vi "001 planta emotelladora.vi"() -> ()   [LabVIEW 2019]
panel:
  in  "pos ampolla plena":dbl(slide) scale=0.0..100.0
  out "Horizontal Pointer Slide":dbl(slide) scale=0.0..100.0
  in  "dispensador":dbl(slide) scale=0.0..10.0
  out "Slide":dbl(slide) scale=0.0..10.0
  in  "pos ampolla buida":dbl(slide) scale=0.0..100.0
  out "Horizontal Pointer Slide 2":dbl(slide) scale=0.0..100.0
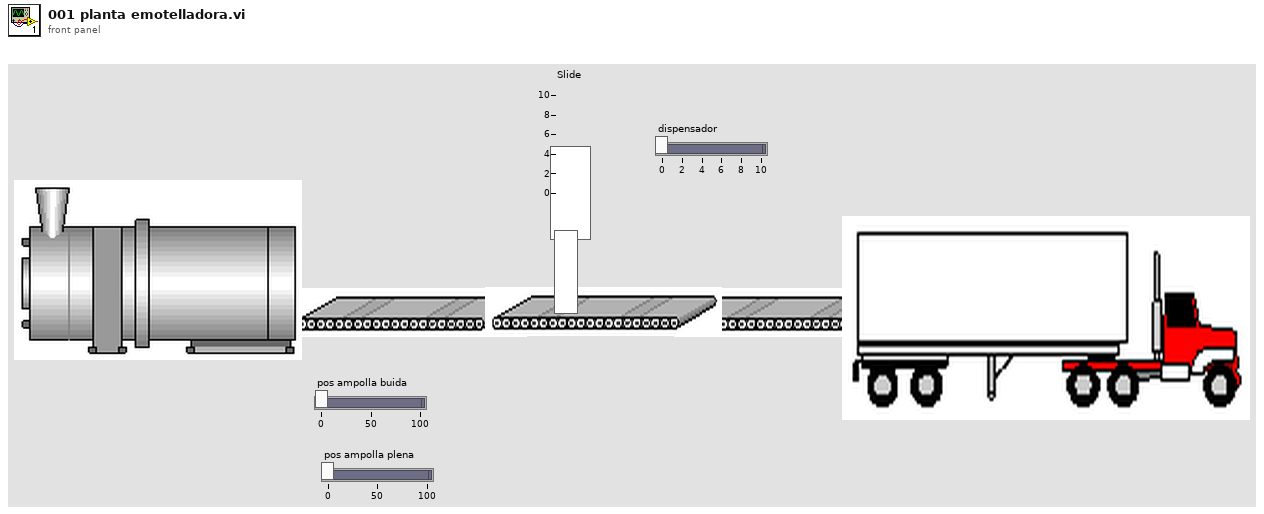
[diagram p1: front panel]
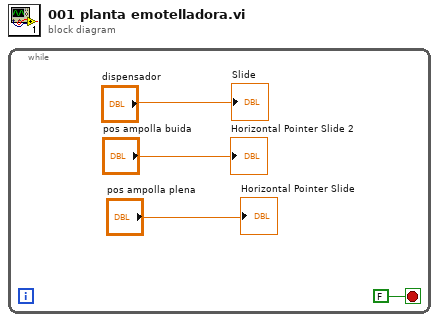
[diagram p0: block diagram]
diagram:
  n1 = while {
    stop <- FALSE stop-if-true
    "Horizontal Pointer Slide 2" <- "pos ampolla buida"
    "Slide" <- "dispensador"
    "Horizontal Pointer Slide" <- "pos ampolla plena"
  }
